vi "Create 3D Cylinder.vi"(1 "Radius":sgl, 2 "Height":sgl, 3 "Color":T1, 4 "Name":string) -> (0 "Scene:New Object":refnum<vi>)   [LabVIEW 2010]
uses:
  <vilib>/picture/3D Picture Control/NI_3D Picture Control.lvlib
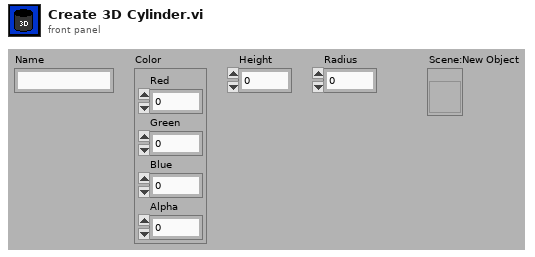
[diagram p1: front panel]
types:
  T1 = cluster{"Red":sgl, "Green":sgl, "Blue":sgl, "Alpha":sgl}
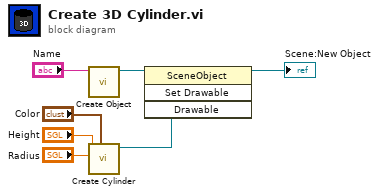
[diagram p0: block diagram]
diagram:
  n1 = call <vilib>:"Create Object.vi"("Name"="Name") -> ("Scene:New Object"=w6:refnum<vi>)  [unwired: 9 in, 1 out]
  n2 = call <vilib>:"Create Cylinder.vi"("Color"="Color", "Radius"="Radius", "Height"="Height") -> ("New Cylinder Refnum"=w5:refnum<vi>)  [unwired: 7 in, 1 out]
  n3 = invoke class="SceneObject" method="Set Drawable"(reference=w6, "Drawable"=w5) -> (reference out=→"Scene:New Object":refnum<vi>)  [unwired: 2 in, 3 out]
